vi "mVToScl.vi"(3 "all":bool, 4 "Length":u8, 5 "1st ch#":u8, 6 "Ain[]":i32[](array[numeric])=[8545, 7019, 6409, 6714, 7324, 8545, 7629, 6409, 305, 610, -4273, -3663, -3358, 0, 2747, -3053, 7324, 7935, 7324, 3967, 8545, 8240, 7629, 5493, 4578, 2747, 1526, 610, 305, 3052, 2441, -10000001, 3052, 1831, 610, 1831, 9990540, 2747, 2747, 9900818, 503845, 8004761, 7019, 3967, 6714, 5798, 5493, 3357]) -> (0 "Scale":dbl[](array[numeric])=[427.25, 701.9000000000001, 64.09, 671.4000000000001, 366.20000000000005, 854.5, 76.29, 640.9000000000001, 30.5, 61.0, 0.0, 0.0, 0.0, 0.0, 27.47, 0.0, 3662.0, 3967.5, 3662.0, 19835.0, 427.25, 4120.0, 3814.5, 2746.5, 2289.0, 549.4, 763.0, 305.0, nan, nan, 0.7323, 0.40240000000000004, nan, 915.5, 122.0, 183.10000000000002, 999054.0, 1373.5, 0.6988000000000001, 99008.18000000001, 100769.0, 800476.1000000001, nan, nan, nan, nan, nan, nan] format="%.2f")   [LabVIEW 2011]
uses:
  Globals/SysGlbs.vi
panel:
  out "?":i32=47
  in  "Umax":u32=100
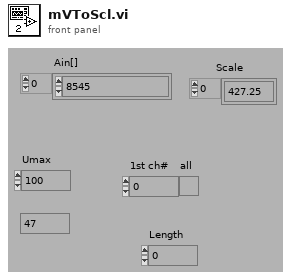
[diagram p1: front panel]
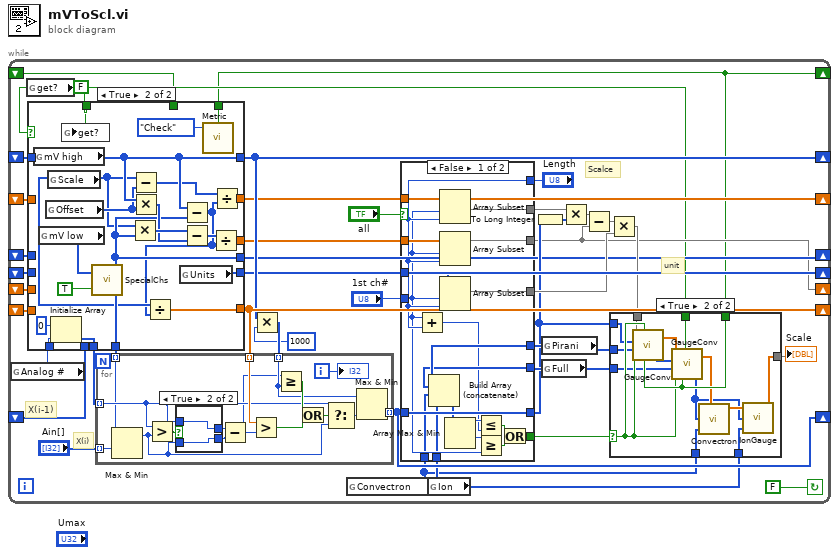
[diagram p0: block diagram]
diagram:
  n1 = while {
    shift-left: _ -> [w3]
    shift-right: [w2] -> _
    shift-left: _ -> [w9]
    shift-right: [w10] -> _
    shift-left: _ -> [w33]
    shift-right: [w8] -> _
    shift-left: _ -> [w32]
    shift-right: [w37] -> _
    shift-left: _ -> [w40]
    shift-right: [w23] -> _
    shift-left: _ -> [w41]
    shift-right: [w27] -> _
    shift-left: _ -> [w42]
    shift-right: [w22] -> _
    shift-left: _ -> [w31]
    shift-right: [w36] -> _
    stop <- FALSE continue-if-true
    w4 = FALSE
    # "X(i)"
    # "X(i-1)"
    # "unit"
    # "Scalce"
    n2 = global read "SysGlbs.vi" "Analog #"() -> (w29:u32)
    n3 = global read "SysGlbs.vi" "get?"() -> (w30:bool)
    n4 = case shown="True" w30 {
      tunnel: [w110 w128] -> w22
      tunnel: [w111 w125] -> w36
      tunnel: w31 -> [w111 _]
      tunnel: w42 -> [w110 _]
      tunnel: [w109 w132] -> w27
      tunnel: w41 -> [w109 _]
      tunnel: w40 -> [w108 _]
      tunnel: [w108 w130] -> w39
      tunnel: [w107 w116] -> w37
      tunnel: w32 -> [w107 _]
      tunnel: [w106 w123] -> w13
      tunnel: w33 -> [w106 _]
      tunnel: w29 -> [_ w129]
      tunnel: w4 -> [_ w126]
      tunnel: [w105 w118] -> w11
      tunnel: [w105 w118] -> w10
      tunnel: w9 -> [w105 _]
      tunnel: [w104 w112] -> w2
      tunnel: w3 -> [w104 _]
      frame False {
      }
      frame True {
        n5 = global read "SysGlbs.vi" "mV high"() -> (w125:i32[])
        n6 = global read "SysGlbs.vi" "mV low"() -> (w127:i32[])
        n7 = global read "SysGlbs.vi" "Offset"() -> (w124:i32[])
        n8 = global read "SysGlbs.vi" "Scale"() -> (w115:i32[])
        n9 = Initialize Array(0, w129) -> (w130:i32[])
        n10 = global write "SysGlbs.vi" "get?"(w126) -> ()
        n11 = call "SpecialChs.vi"("Ain?"=TRUE, "mV low"=w127) -> ("mV low New"=w118:i32[])
        n12 = Multiply(x=w115, y=w118) -> (x*y=w122:i32[])
        n13 = Subtract(x=w115, y=w124) -> (x-y=w119:i32[])
        n14 = Multiply(x=w125, y=w124) -> (x*y=w121:i32[])
        n15 = global read "SysGlbs.vi" "Units"() -> (w128:u8[])
        n16 = Subtract(x=w125, y=w118) -> (x-y=w114:i32[])
        n17 = Divide(x=w115, y=w114) -> (x/y=w116:dbl[])
        n18 = Subtract(x=w122, y=w121) -> (x-y=w120:i32[])
        n19 = call "Metric.vi"("Action"=enum16{"Init", "Check"}."Check") -> ("Metric?"=w112:bool)  [unwired: 4 in]
        n20 = Divide(x=w120, y=w114) -> (x/y=w123:dbl[])
        n21 = Divide(x=w119, y=w114) -> (x/y=w132:dbl[])
      }
    }
    n22 = Multiply(x=w36, y=1000) -> (x*y=w35:i32[])
    n23 = for {
      tunnel: w39 -> [w91] mode=indexing
      tunnel: [w99] -> w23 mode=indexing
      tunnel: "Ain[]" -> [w85] mode=indexing
      tunnel: w37 -> [w94] mode=indexing
      tunnel: w35 -> [w95] mode=indexing
      tunnel: w11 -> [w86] mode=indexing
      i -> [w93]
      n24 = Max & Min(x=w86, y=w85) -> (max(x,y)=w84:i32)  [unwired: 1 out]
      n25 = Greater?(x=w91, y=w84) -> (0:w92:bool)
      n26 = case shown="True" w92 {
        tunnel: w91 -> [w101 w103]
        tunnel: w84 -> [w100 w102]
        tunnel: [w100 w103] -> w90
        tunnel: [w101 w102] -> w89
        frame False {
        }
        frame True {
        }
      }
      n27 = Subtract(x=w90, y=w89) -> (x-y=w87:i32)
      n28 = Greater?(x=w94, y=w87) -> (0:w88:bool)
      n29 = Greater Or Equal?(x=w87, y=w95) -> (x >= y?=w97:bool)
      n30 = Or(x=w97, y=w88) -> (x .or. y?=w96:bool)
      n31 = Select(t=w91, s=w96, f=w84) -> (s? t:f=w98:i32)
      n32 = Max & Min(x=w95, y=w98) -> (min(x,y)=w99:i32)  [unwired: 1 out]
      "?" <- w93
    }
    n33 = global read "SysGlbs.vi" "Convectron"() -> (w6:i32[])
    n34 = global read "SysGlbs.vi" "Ion"() -> (w7:i32[])
    n35 = global read "SysGlbs.vi" "Pirani"() -> (w16:i32[])
    n36 = global read "SysGlbs.vi" "Full"() -> (w17:i32[])
    n37 = case shown="False" "all" {
      selector: "all" -> [_ w80]
      tunnel: w27 -> [w78 w83]
      tunnel: [w77 w83] -> w26
      tunnel: "1st ch#" -> [w65 _]
      tunnel: "Length" -> [w72 _]
      tunnel: w23 -> [w73 w82]
      tunnel: [w73 w82] -> w15
      tunnel: w22 -> [w76 w81]
      tunnel: [w75 w81] -> w21
      tunnel: w13 -> [w74 w79]
      tunnel: w16 -> [w71 _]
      tunnel: w17 -> [w70 _]
      tunnel: [w62 w80] -> w18
      tunnel: [w61 w79] -> w8
      tunnel: w6 -> [w60 _]
      tunnel: w7 -> [w59 _]
      frame False {
        n38 = Add(x=w65, y=w72) -> (x+y=w66:u8)
        n39 = Build Array (concatenate)(w71, w70, w60, w59) -> (w69:i32[])
        n40 = Array Subset(array=w78, index=w65, length=w72) -> (w77:dbl[])
        n41 = Array Subset(array=w74, index=w65, length=w72) -> (w61:dbl[])
        n42 = Array Subset(array=w76, index=w65, length=w72) -> (w75:u8[])
        n43 = Array Max & Min(array=w69) -> (max value=w67:i32, min value=w68:i32)  [unwired: 2 out]
        n44 = Less Or Equal?(x=w67, y=w66) -> (x <= y?=w64:bool)
        n45 = Greater Or Equal?(x=w68, y=w65) -> (x >= y?=w63:bool)
        n46 = Or(x=w64, y=w63) -> (x .or. y?=w62:bool)
      }
      frame True {
      }
    }
    n47 = To Long Integer(number=w15) -> (32bit integer=w20:i32[])
    n48 = Multiply(x=w26, y=w20) -> (x*y=w14:dbl[])
    n49 = Subtract(x=w14, y=w8) -> (x-y=w12:dbl[])
    n50 = Multiply(x=w12, y=w21) -> (x*y=w19:dbl[])
    n51 = case shown="True" w18 {
      selector: w18 -> [_ w55]
      tunnel: [w43 w47] -> w5
      tunnel: w2 -> [_ w56]
      tunnel: w19 -> [w43 w53]
      tunnel: w17 -> [_ w54]
      tunnel: w16 -> [_ w52]
      tunnel: w15 -> [_ w51]
      tunnel: w6 -> [_ w49]
      tunnel: w7 -> [_ w46]
      tunnel: w4 -> [_ w44]
      frame False {
      }
      frame True {
        n52 = call "GaugeConv.vi"("mbar?"=w56, "Pirani?"=w55, "V-To-P?"=w55, "Index"=w52, "Voltage"=w51, "Press"=w53) -> ("Voltage out"=w57:u32[], "Press out"=w58:dbl[])
        n53 = call "GaugeConv.vi"("mbar?"=w56, "Pirani?"=w44, "V-To-P?"=w55, "Index"=w54, "Voltage"=w57, "Press"=w58) -> ("Voltage out"=w45:u32[], "Press out"=w50:dbl[])
        n54 = call "Convectron.vi"("Index"=w49, "Voltage"=w45, "Scale"=w50) -> ("Scale out"=w48:dbl[])  [unwired: 2 in]
        n55 = call "IonGauge.vi"("Index"=w46, "Voltage"=w45, "Scale"=w48) -> ("Scale out"=w47:dbl[])  [unwired: 2 in]
      }
    }
    "Scale" <- w5
  }
